vi "Picture.vi"(0 "path to BMP file":path, 1 "XML File Path":path, 2 "In":refnum<vi>, 3 "Out":refnum<vi>) -> ()   [LabVIEW 2010]
uses:
  <vilib>/xml/NI_XML.lvlib
  C:/Program Files (x86)/National Instruments/LabVIEW 2010/resource/objmgr/DOMUserDefRef.rc
panel:
  out "Boolean":bool caption="out[0]"
  out "Boolean 3":bool caption="in[1]"
  out "Boolean 2":bool caption="in[0]"
  out "?":picture
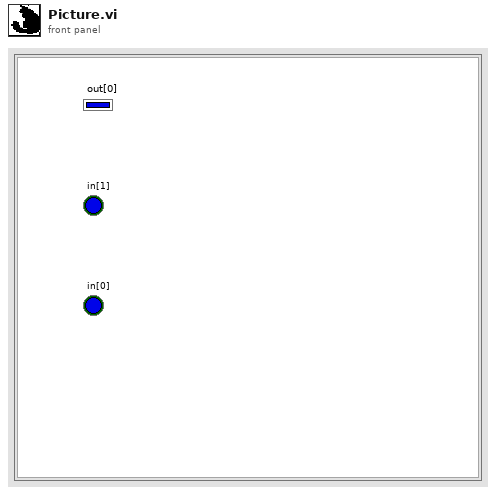
[diagram p1: front panel]
types:
  T1 = typedef "imagedata.ctl" = cluster{"image type":i32, "image depth":i32, "image":u8[], "mask":u8[], "colors":u32[], "Rectangle":cluster{"left":i16, "top":i16, "right":i16, "bottom":i16}}
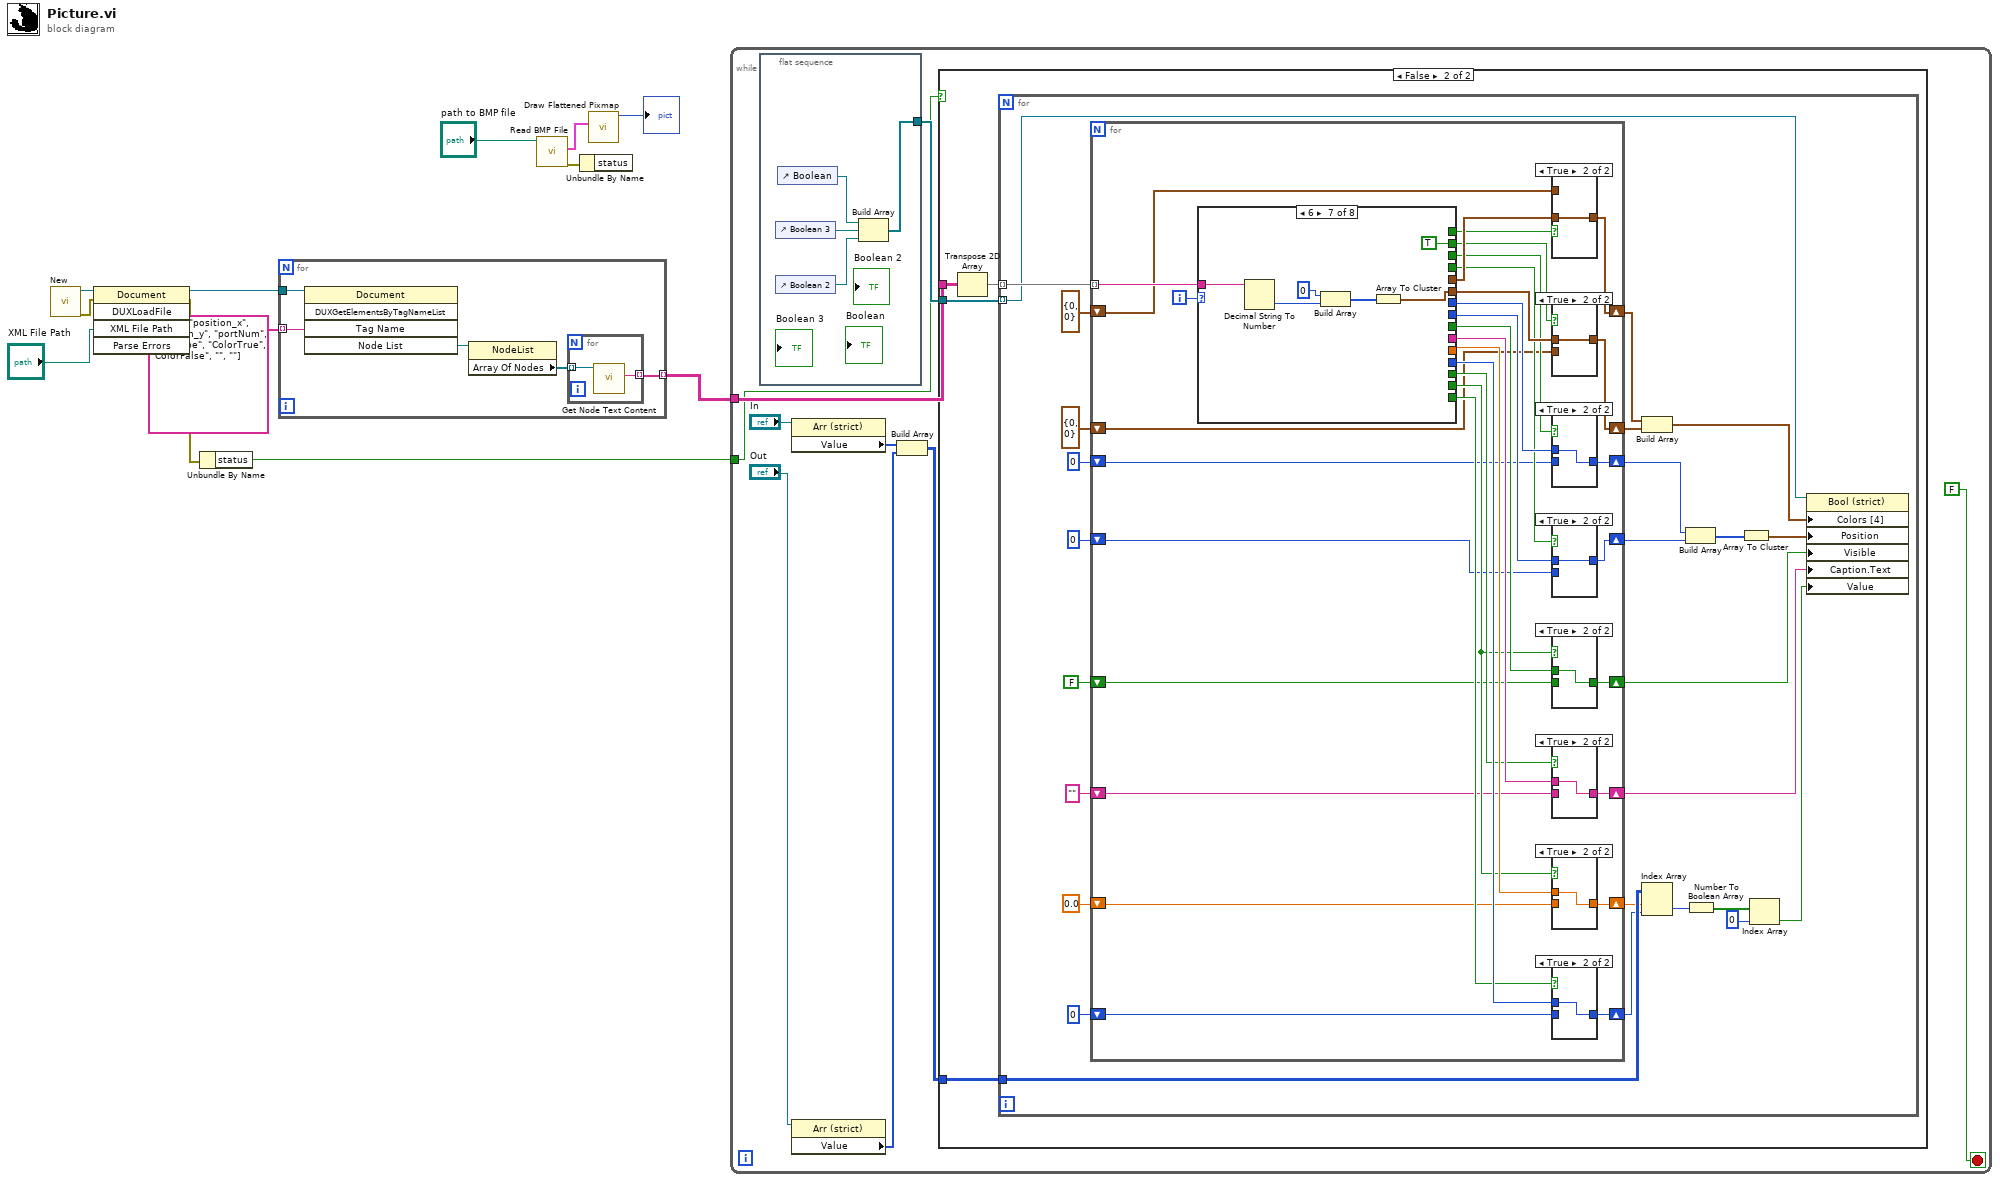
[diagram p0: block diagram]
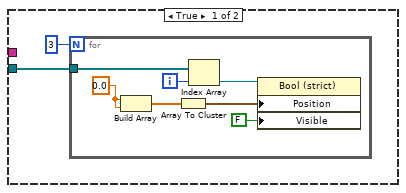
[diagram p2: hidden frame]
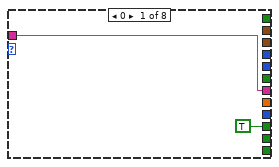
[diagram p11: hidden frame]
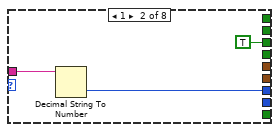
[diagram p12: hidden frame]
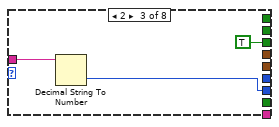
[diagram p13: hidden frame]
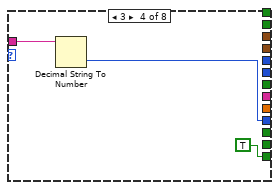
[diagram p14: hidden frame]
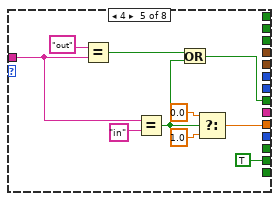
[diagram p15: hidden frame]
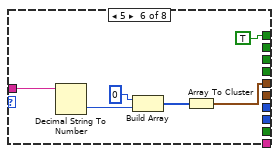
[diagram p16: hidden frame]
diagram:
  n1 = call <vilib>:"New.vi"() -> ("error out"=w9:errorcluster, "DOM document out"=w10:refnum<k20>)  [unwired: 8 in]
  n2 = invoke class="Document" method="DUXLoadFile"(reference=w10, error in=w9, "XML File Path"="XML File Path") -> (reference out=w5:refnum<k20>, error out=w2:errorcluster)  [unwired: 2 in, 3 out]
  n3 = Unbundle By Name(w2) -> ("status"=w1:bool)
  n4 = for {
    tunnel: string[] ["title", "position_x", "position_y", "portNum", "portType", "ColorTrue", "ColorFalse", "", ""] -> [w15] mode=indexing
    tunnel: [w14] -> w6 mode=indexing
    tunnel: w5 -> [w13]
    n5 = invoke class="Document" method="DUXGetElementsByTagNameList"(reference=w13, "Tag Name"=w15) -> ("Node List"=w17:refnum<k20>)  [unwired: 3 in, 4 out]
    n6 = property class="NodeList"(reference=w17) -> ("Array Of Nodes"=w16:refnum<k20>[])  [unwired: 1 in, 2 out]
    n7 = for {
      tunnel: w16 -> [w19] mode=indexing
      tunnel: [w18] -> w14 mode=indexing
      n8 = call <vilib>:"Get Node Text Content.vi"("node in"=w19) -> ("node text"=w18:string)  [unwired: 8 in, 2 out]
    }
  }
  n9 = call <vilib>:"Read BMP File.vi"("path to BMP file"="path to BMP file") -> ("error out"=w12:errorcluster, "image data"=w11:T1)  [unwired: 8 in, 1 out]
  n10 = Unbundle By Name(w12) -> ()  [unwired: 1 out]
  n11 = call <vilib>:"Draw Flattened Pixmap.vi"("image data"=w11) -> ("new picture"=→"?":picture)  [unwired: 8 in]
  n12 = while {
    tunnel: w6 -> [w26]
    tunnel: w1 -> [w25]
    stop <- FALSE stop-if-true
    n13 = flat-sequence {
      tunnel: [w30] -> w27
      frame #0 {
        n14 = control-ref of="Boolean 3"() -> (w31:refnum<vi>)
        n15 = control-ref of="Boolean 2"() -> (w29:refnum<vi>)
        n16 = control-ref of="Boolean"() -> (w32:refnum<vi>)
        n17 = Build Array(w32, w31, w29) -> (w30:refnum<vi>[])
      }
    }
    n18 = property class="Arr (strict)"(reference="In") -> ("Value"=w23:i8[])  [unwired: 1 in, 2 out]
    n19 = property class="Arr (strict)"(reference="Out") -> ("Value"=w21:i8[])  [unwired: 1 in, 2 out]
    n20 = Build Array(w23, w21) -> (w20:i8[][])
    n21 = case shown="False" w25 {
      tunnel: w27 -> [w33 w45]
      tunnel: w20 -> [_ w44]
      tunnel: w26 -> [_ w42]
      frame True {
        n22 = for {
          N: 3 -> [_]
          tunnel: w33 -> [w36]
          i -> [w35]
          w38 = 0.0 ("element")
          n23 = Build Array(w38, w38) -> (w41:dbl[])
          n24 = Array To Cluster(array=w41) -> (cluster=w39:cluster{"[0]":dbl, "[1]":dbl})
          n25 = Index Array(array=w36, index=w35) -> (element=w37:refnum<vi>)
          n26 = property on="Property Node" class="Bool (strict)"(reference=w37, "Position"=w39, "Visible"=FALSE) -> ()  [unwired: 1 in, 2 out]
        }
      }
      frame False {
        n27 = Transpose 2D Array(2D array=w42) -> (transposed array=w43:string[][])
        n28 = for {
          tunnel: w43 -> [w63] mode=indexing
          tunnel: w45 -> [w58] mode=indexing
          tunnel: w44 -> [w68]
          n29 = for {
            tunnel: w63 -> [w104] mode=indexing
            shift-right: [w86] -> w57
            shift-left: "" ("node text") -> [w87]
            shift-right: [w84] -> w62
            shift-left: 0 ("Numeric") -> [w85]
            shift-right: [w82] -> w61
            shift-left: 0 ("Numeric") -> [w83]
            shift-right: [w80] -> w60
            shift-left: 0 ("Numeric") -> [w81]
            shift-right: [w78] -> w59
            shift-left: 0.0 ("f") -> [w79]
            shift-right: [w76] -> w55
            shift-left: cluster{"[0]":i32, "[1]":i32} {"[0]"=0, "[1]"=0} ("Cluster") -> [w77]
            shift-right: [w74] -> w54
            shift-left: cluster{"[0]":i32, "[1]":i32} {"[0]"=0, "[1]"=0} ("Cluster") -> [w75]
            shift-right: [w72] -> w56
            shift-left: FALSE ("Boolean 4") -> [w73]
            i -> [w96]
            n30 = case shown="6" w96 {
              tunnel: w104 -> [w121 w125 w128 w131 w132 w147 w153 _]
              tunnel: [w121 _ _ _ _ _ _ _] -> w97
              tunnel: [_ w124 _ _ _ _ _ _] -> w103
              tunnel: [_ _ w127 _ _ _ _ _] -> w102
              tunnel: [_ _ _ w130 _ _ _ _] -> w101
              tunnel: [_ _ _ _ w139 _ _ _] -> w100
              tunnel: [_ _ _ _ _ w144 _ _] -> w99
              tunnel: [_ _ _ _ _ _ w148 _] -> w98
              tunnel: [TRUE _ _ _ _ _ _ _] -> w95
              tunnel: [_ _ _ _ TRUE _ _ _] -> w88
              tunnel: [_ _ _ _ _ TRUE _ _] -> w94
              tunnel: [_ _ _ _ _ _ TRUE _] -> w93
              tunnel: [_ TRUE _ _ _ _ _ _] -> w92
              tunnel: [_ _ TRUE _ _ _ _ _] -> w91
              tunnel: [_ _ _ TRUE _ _ _ _] -> w90
              tunnel: [_ _ _ _ w137 _ _ _] -> w89
              frame 0 {
              }
              frame 1 {
                n31 = Decimal String To Number(string=w125) -> (number=w124:i32)  [unwired: 2 in, 1 out]
              }
              frame 2 {
                n32 = Decimal String To Number(string=w128) -> (number=w127:i32)  [unwired: 2 in, 1 out]
              }
              frame 3 {
                n33 = Decimal String To Number(string=w131) -> (number=w130:i32)  [unwired: 2 in, 1 out]
              }
              frame 4 {
                n34 = Equal?(x="out", y=w132) -> (x = y?=w134:bool)
                n35 = Equal?(x=w132, y="in") -> (x = y?=w133:bool)
                n36 = Or(x=w134, y=w133) -> (x .or. y?=w137:bool)
                n37 = Select(t=0.0, s=w133, f=1.0) -> (s? t:f=w139:dbl)
              }
              frame 5 {
                n38 = Decimal String To Number(string=w147) -> (number=w142:i32)  [unwired: 2 in, 1 out]
                n39 = Build Array(0 ("element"), w142) -> (w145:i32[])
                n40 = Array To Cluster(array=w145) -> (cluster=w144:cluster{"[0]":i32, "[1]":i32})
              }
              frame 6 {
                n41 = Decimal String To Number(string=w153) -> (number=w149:i32)  [unwired: 2 in, 1 out]
                n42 = Build Array(0 ("element"), w149) -> (w151:i32[])
                n43 = Array To Cluster(array=w151) -> (cluster=w148:cluster{"[0]":i32, "[1]":i32})
              }
              frame -1, Default {
              }
            }
            n44 = case shown="True" w94 {
              tunnel: w77 -> [w109 _]
              tunnel: w99 -> [_ w110]
              tunnel: [w109 w110] -> w76
              frame False {
              }
              frame True {
              }
            }
            n45 = case shown="True" w93 {
              tunnel: w75 -> [w107 _]
              tunnel: w98 -> [_ w108]
              tunnel: [w107 w108] -> w74
              frame False {
              }
              frame True {
              }
            }
            n46 = case shown="True" w92 {
              tunnel: w85 -> [w117 _]
              tunnel: w103 -> [_ w118]
              tunnel: [w117 w118] -> w84
              frame False {
              }
              frame True {
              }
            }
            n47 = case shown="True" w91 {
              tunnel: w83 -> [w115 _]
              tunnel: w102 -> [_ w116]
              tunnel: [w115 w116] -> w82
              frame False {
              }
              frame True {
              }
            }
            n48 = case shown="True" w88 {
              tunnel: w73 -> [w105 _]
              tunnel: w89 -> [_ w106]
              tunnel: [w105 w106] -> w72
              frame False {
              }
              frame True {
              }
            }
            n49 = case shown="True" w95 {
              tunnel: w87 -> [w119 _]
              tunnel: w97 -> [_ w120]
              tunnel: [w119 w120] -> w86
              frame False {
              }
              frame True {
              }
            }
            n50 = case shown="True" w88 {
              tunnel: w79 -> [w111 _]
              tunnel: w100 -> [_ w112]
              tunnel: [w111 w112] -> w78
              frame False {
              }
              frame True {
              }
            }
            n51 = case shown="True" w90 {
              tunnel: w81 -> [w113 _]
              tunnel: w101 -> [_ w114]
              tunnel: [w113 w114] -> w80
              frame False {
              }
              frame True {
              }
            }
          }
          n52 = Build Array(w55, w54) -> (w69:cluster{"[0]":i32, "[1]":i32}[])
          n53 = Index Array(array=w68, index (row)=w59, index (col)=w60) -> (element=w64:i8)
          n54 = Build Array(w62, w61) -> (w71:i32[])
          n55 = Number To Boolean Array(number=w64) -> (Boolean array=w65:bool[])
          n56 = Array To Cluster(array=w71) -> (cluster=w70:cluster{"[0]":i32, "[1]":i32})
          n57 = Index Array(array=w65, index=0) -> (element=w66:bool)
          n58 = property on="Property Node" class="Bool (strict)"(reference=w58, "Colors [4]"=w69, "Position"=w70, "Visible"=w56, "Caption.Text"=w57, "Value"=w66) -> ()  [unwired: 1 in, 2 out]
        }
      }
    }
  }
